vi "PicoScope5000aExampleRapidBlock.vi"() -> ()   [LabVIEW 2015]
panel:
  in  "Serial Number":string
  in  "Open using Serial Number":bool
  in  "Resolution":i32(ring)=4 items=["8-bit", "12-bit", "14-bit", "15-bit (max. 2 ch.)", "16-bit (max. 1 ch.)"]
  in  "PS5X4XA/B\nUSB Powered":bool=TRUE
  in  "Trigger Settings":T1={"Trigger Enabled"=TRUE, "Trigger Source"=enum."Channel A", "Trigger Threshold (16-bit counts)"=16384, "Trigger Direction"=2, "Trigger Delay (samples)"=0, "Auto Trigger Time (ms)"=0} {"Trigger Direction" items=["Rising"=2, "Falling"=3]}
  in  "Channel A Settings":T2={"Enabled"=TRUE, "Coupling"=1, "Range"=6, "Analogue Offset"=0.0} {"Range" items=["10 mV", "20 mV", "50 mV", "100 mV", "200 mV", "500 mV", "1 V", "2 V", "5 V", "10 V", "20 V", "50 V ", "100 V"]; "Coupling" items=["AC", "DC"]}
  in  "Rapid Block Acquisition Settings":T3={"preTriggerSamples"=0, "postTriggerSamples"=1024, "timebase"=10, "Four Channel Device"=FALSE, "Number of Captures"=100}
  out "Capture Complete":bool
  in  "Run":bool
  out "Channel A":i16[][](graph)
  in  "Capture Index":i16 min=0
  in  "stop":bool
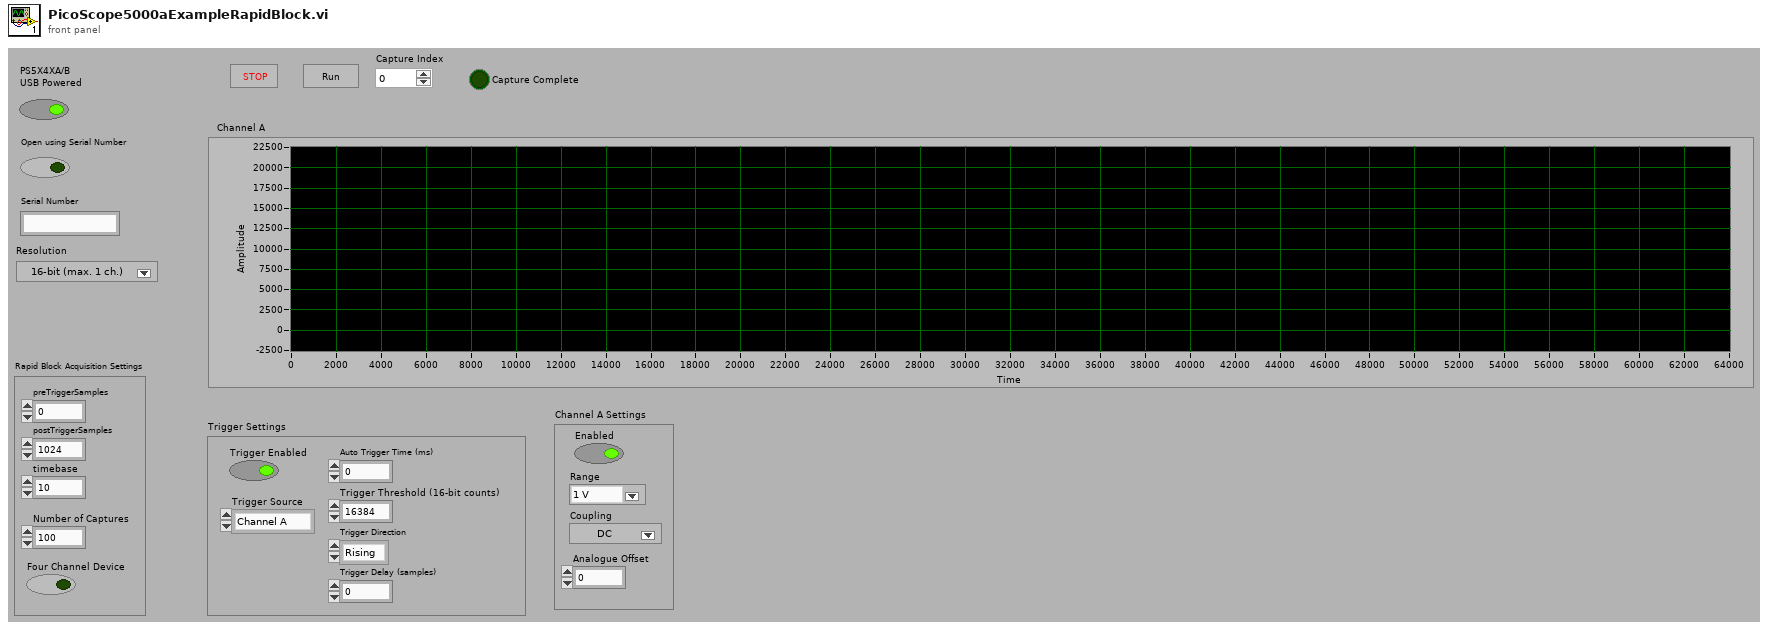
[diagram p1: front panel]
types:
  T1 = cluster{"Trigger Enabled":bool, "Trigger Source":enum16{"Channel A", "Channel B", "Channel C", "Channel D", "Ext."}, "Trigger Threshold (16-bit counts)":i16, "Trigger Direction":u16, "Trigger Delay (samples)":u32, "Auto Trigger Time (ms)":i16}
  T2 = cluster{"Enabled":bool, "Coupling":i16, "Range":u16, "Analogue Offset":sgl}
  T3 = cluster{"preTriggerSamples":u32, "postTriggerSamples":u32, "timebase":u32, "Four Channel Device":bool, "Number of Captures":u32}
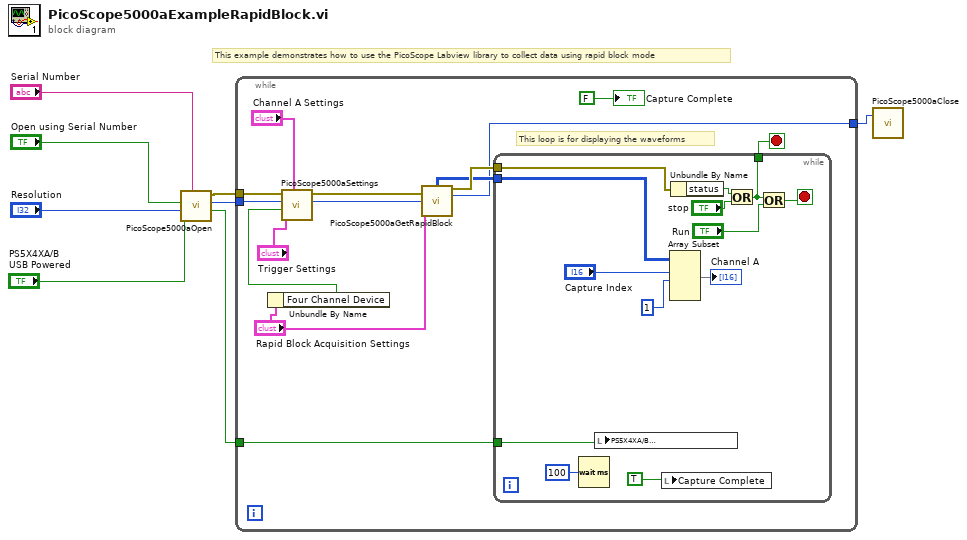
[diagram p0: block diagram]
diagram:
  # "This example demonstrates how to use the PicoScope Labview library to collect data using rapid block mode"
  n1 = call "PicoScope5000aOpen.vi"("Serial Number"="Serial Number", "USB Powered Selection"="PS5X4XA/B\nUSB Powered", "Resolution"="Resolution", "Use Serial Number"="Open using Serial Number") -> ("USB Powered Indication"=w4:bool, "handle"=w6:i16, "error out"=w7:errorcluster)  [unwired: 2 in, 1 out]
  n2 = while {
    tunnel: [w18] -> w8
    tunnel: w7 -> [w13]
    tunnel: w6 -> [w12]
    tunnel: w4 -> [w11]
    stop <- w22 stop-if-true
    # "This loop is for displaying the waveforms"
    n3 = Unbundle By Name("Rapid Block Acquisition Settings") -> ("Four Channel Device"=w9:bool)
    n4 = call "PicoScope5000aSettings.vi"("Channel A Settings"="Channel A Settings", "Trigger Settings"="Trigger Settings", "Four Channel Device?"=w9, "handle in"=w12, "error in"=w13) -> ("handle out"=w17:i16, "error out"=w16:errorcluster)  [unwired: 5 in]
    n5 = call "PicoScope5000aGetRapidBlock.vi"("error in"=w16, "handle in"=w17, "Rapid Block Acquisition Settings"="Rapid Block Acquisition Settings") -> ("Channel A Buffer"=w19:i16[][], "error out"=w20:errorcluster, "handle out"=w18:i16)  [unwired: 7 in, 3 out]
    n6 = while {
      tunnel: [w32] -> w22
      tunnel: w19 -> [w27]
      tunnel: w20 -> [w26]
      tunnel: w11 -> [w23]
      stop <- w31 stop-if-true
      n7 = Wait (ms)(milliseconds to wait=u32 100) -> ()  [unwired: 1 out]
      n8 = local write "PS5X4XA/B\nUSB Powered"(w23) -> ()
      n9 = local write "Capture Complete"(TRUE ("Capture Complete")) -> ()
      n10 = Array Subset(array=w27, index (row)="Capture Index", length (row)=1 ("length")) -> (→"Channel A":i16[][])  [unwired: 2 in]
      n11 = Unbundle By Name(w26) -> ("status"=w25:bool)
      n12 = Or(x=w25, y="stop") -> (x .or. y?=w32:bool)
      n13 = Or(x=w32, y="Run") -> (x .or. y?=w31:bool)
    }
    "Capture Complete" <- FALSE ("Capture Complete")
  }
  n14 = call "PicoScope5000aClose.vi"("handle"=w8) -> ()  [unwired: 2 in, 1 out]
